vi "Control Panel.vi"(8 "error in":errorcluster, 11 "Varian Magnet.lvclass":refnum<class "Varian Magnet.lvclass">) -> (0 "error out":errorcluster, 3 "Varian Magnet.lvclass out":refnum<class "Varian Magnet.lvclass">)   [LabVIEW 2009, in "Varian Magnet.lvclass"]
uses:
  Varian Magnet.lvclass
panel:
  in  "Control Voltage":enum16{"Please Select a Value", "30V", "40V"}(ring)=enum."40V"
  out "At field and stable?":bool
  in  "Go to field (stable)":bool
  in  "Read current field":bool
  in  "Go to field (immediately)":bool
  out "Current field":dbl[unit]
  in  "Desired field":dbl[unit]
  in  "stop":bool
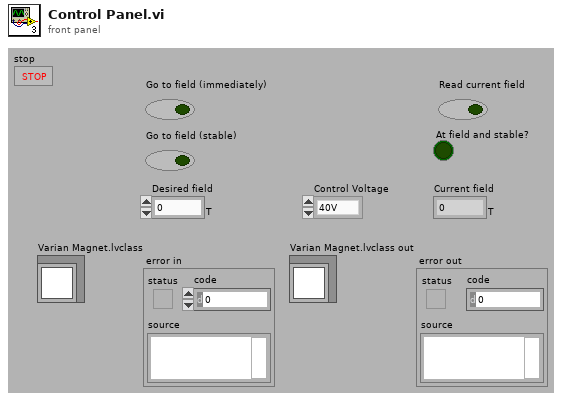
[diagram p1: front panel]
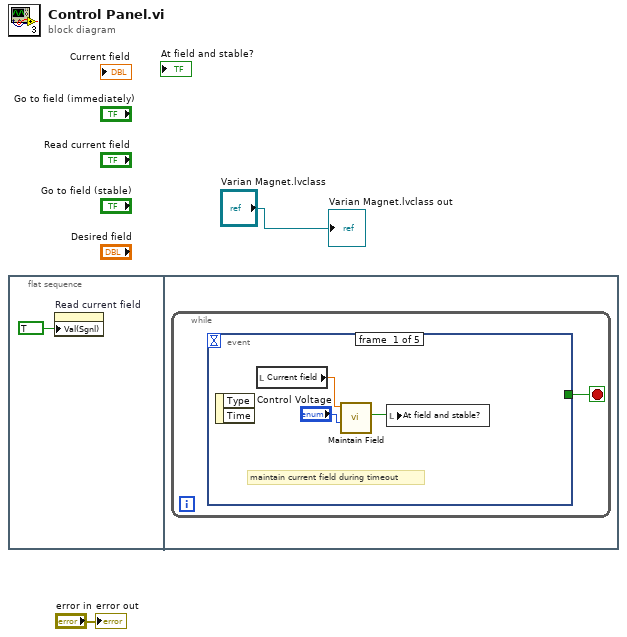
[diagram p0: block diagram]
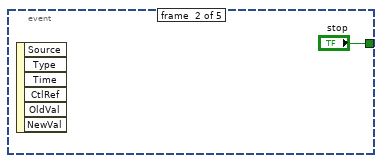
[diagram p2: hidden frame]
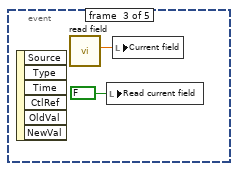
[diagram p3: hidden frame]
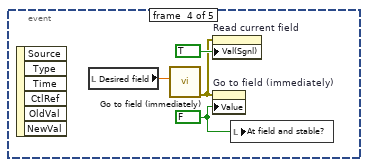
[diagram p4: hidden frame]
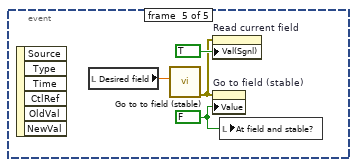
[diagram p5: hidden frame]
diagram:
  n1 = flat-sequence {
    frame #0 {
      n2 = property on="Read current field" class="Bool (strict)"("Val(Sgnl)"=TRUE ("Value (Signaling)")) -> ()  [unwired: 2 in, 2 out]
    }
    frame #1 {
      n3 = while {
        stop <- w4 stop-if-true
        n4 = event shown="[4] \"Go to field (stable)\": Value Change" {
          selector: _ -> [_ _ _ _ _]
          dyn-events: _ -> [_ _ _ _ _]
          timeout: _ -> [_ _ _ _ _]
          tunnel: [_ "stop" _ _ _] -> w4
          event #0 {
            # "maintain current field during timeout"
            n5 = event-data() -> ()  [unwired: 3 out]
            n6 = local read "Current field"() -> (w6:dbl[unit])
            n7 = call "Maintain Field.vi"("Enum"="Control Voltage", "Desired field"=w6) -> ("At field and stable?"=w5:bool)  [unwired: 8 in, 1 out]
            n8 = local write "At field and stable?"(w5) -> ()
          }
          event #1 {
            n9 = event-data() -> ()  [unwired: 7 out]
          }
          event #2 {
            n10 = event-data() -> ()  [unwired: 7 out]
            n11 = call "read field.vi"() -> ("Current field (T)"=w9:dbl[unit])  [unwired: 1 in, 10 out]
            n12 = local write "Read current field"(FALSE ("Read current field")) -> ()
            n13 = local write "Current field"(w9) -> ()
          }
          event #3 {
            w11 = FALSE ("Go to field")
            n14 = event-data() -> ()  [unwired: 7 out]
            n15 = local read "Desired field"() -> (w14:dbl[unit])
            n16 = call "Go to field (immediately).vi"("Desired field (T)"=w14) -> ("error out"=w12:errorcluster)  [unwired: 1 in, 9 out]
            n17 = property on="Read current field" class="Bool (strict)"(error in=w12, "Val(Sgnl)"=TRUE ("Value (Signaling)")) -> ()  [unwired: 1 in, 2 out]
            n18 = property on="Go to field (immediately)" class="Bool (strict)"(error in=w12, "Value"=w11) -> ()  [unwired: 1 in, 2 out]
            n19 = local write "At field and stable?"(w11) -> ()
          }
          event #4 {
            w15 = FALSE ("Go to field (stable)")
            n20 = event-data() -> ()  [unwired: 7 out]
            n21 = local read "Desired field"() -> (w17:dbl[unit])
            n22 = call "Go to to field (stable).vi"("Desired field"=w17) -> ("error out"=w16:errorcluster)  [unwired: 2 in, 8 out]
            n23 = property on="Read current field" class="Bool (strict)"(error in=w16, "Val(Sgnl)"=TRUE ("Value (Signaling)")) -> ()  [unwired: 1 in, 2 out]
            n24 = property on="Go to field (stable)" class="Bool (strict)"(error in=w16, "Value"=w15) -> ()  [unwired: 1 in, 2 out]
            n25 = local write "At field and stable?"(w15) -> ()
          }
        }
      }
    }
  }
  "Varian Magnet.lvclass out" <- "Varian Magnet.lvclass"
  "error out" <- "error in"
